vi "From Serial Form.vi"(6 "Serial Version":T1, 10 "Deserializer in":refnum<class "Deserializer.lvclass">=refnum, 11 "Alicat in":refnum<class "Alicat.lvclass">) -> (0 "error out":errorcluster, 2 "Deserializer out":refnum<class "Deserializer.lvclass">, 3 "Alicat out":refnum<class "Alicat.lvclass">)   [LabVIEW 2014]
uses:
  Controls/Gas.ctl
  Alicat.lvclass
  <userlib>/Serialization/Serializable/Remove Boolean.vi
  <userlib>/Serialization/Serializable/Remove Int16.vi
  <userlib>/Serialization/Serializable/Remove String.vi
  <userlib>/Serialization/Serialization Common/Serial Version.ctl
  <userlib>/Serialization/Deserializer/Deserializer.lvclass
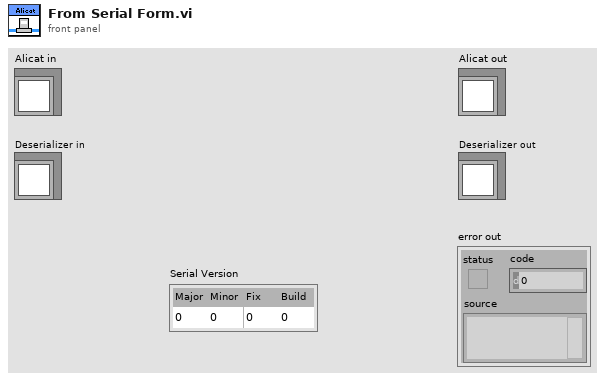
[diagram p1: front panel]
types:
  T1 = typedef "Serialization Common.lvlib/Serial Version.ctl" = cluster{"Major":u16, "Minor":u16, "Fix":u16, "Build":u16}
  T2 = typedef "Alicat.lvlib/Alicat.lvclass/Gas.ctl" = enum16{"Air", "Ar", "CH4", "CO", "CO2", "C2H6", "H2", "He", "N2", "NO", "Ne", "O2", "C3H8", "n-C4H10", "C2H2", "C2H4", "i-C2H10", "Kr", "Xe"}
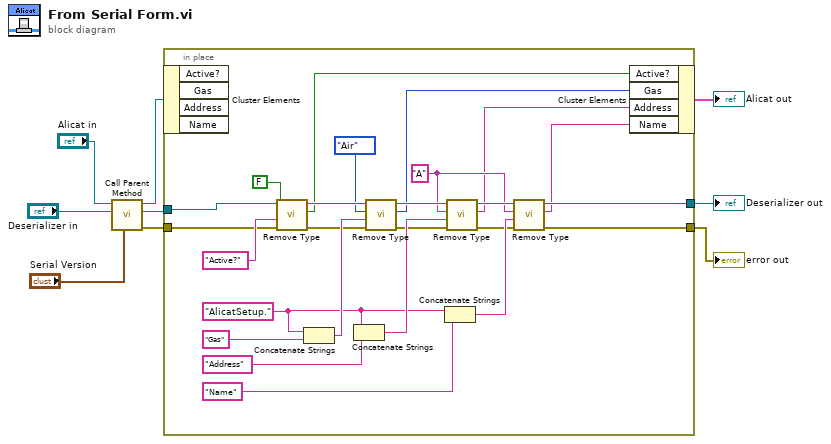
[diagram p0: block diagram]
diagram:
  n1 = call-parent "Call Parent Method"("Serial Version"="Serial Version", "Deserializer in"="Deserializer in", "Serializable in"="Alicat in") -> ("error out"=w5:errorcluster, "Deserializer out"=w6:refnum<class "Deserializer.lvclass">, "Serializable out"=w4:refnum<class "Serializable.lvclass">)  [unwired: 6 in]
  n2 = in-place {
    in-place-border: w6 -> [w34]
    in-place-border: w5 -> [w31]
    in-place-border: [w17] -> w2
    in-place-border: [w16] -> w1
    w14 = "A" ("Default Value")
    w21 = "AlicatSetup."
    n3 = in-place-cluster #1(w4) -> ()  [unwired: 4 out]
    n4 = call-poly <userlib>:"Remove Type.vi"("error in (no error)"=w31, "Name"="Active?", "Default Value"=FALSE, "Deserializer in"=w34) -> ("error out"=w15:errorcluster, "Boolean"=w13:bool, "Deserializer out"=w28:refnum<class "Deserializer.lvclass">)  [unwired: 4 in, 1 out]
    n5 = Concatenate Strings(w21, "Gas" ("string")) -> (w29:string)
    n6 = Concatenate Strings(w21, "Address" ("string")) -> (w24:string)
    n7 = call-poly <userlib>:"Remove Type.vi"("error in (no error)"=w15, "Name"=w29, "Default Value"=Gas."Air" ("AlicatSetup.Gas"), "Deserializer in"=w28) -> ("error out"=w23:errorcluster, "Numeric"=w12:i16, "Deserializer out"=w26:refnum<class "Deserializer.lvclass">)  [unwired: 4 in, 1 out]
    n8 = Concatenate Strings(w21, "Name" ("string")) -> (w19:string)
    n9 = call-poly <userlib>:"Remove Type.vi"("error in (no error)"=w23, "Name"=w24, "Default Value"=w14, "Deserializer in"=w26) -> ("error out"=w18:errorcluster, "String"=w11:string, "Deserializer out"=w22:refnum<class "Deserializer.lvclass">)  [unwired: 4 in, 1 out]
    n10 = call-poly <userlib>:"Remove Type.vi"("error in (no error)"=w18, "Name"=w19, "Default Value"=w14, "Deserializer in"=w22) -> ("error out"=w16:errorcluster, "String"=w10:string, "Deserializer out"=w17:refnum<class "Deserializer.lvclass">)  [unwired: 4 in, 1 out]
    n11 = in-place-cluster #1("Active?"=w13, "Gas"=w12, "Address"=w11, "Name"=w10) -> (→"Alicat out":cluster{})
  }
  "error out" <- w1
  "Deserializer out" <- w2
